vi "Validate Mode.vi"(1 "Mode Array":T1) -> (0 "Mode":i16[](array[numeric]))   [LabVIEW 2019]
uses:
  Version 2/Data Type Defs/Pulse Mode (array).ctl
panel:
  out "Warning":string
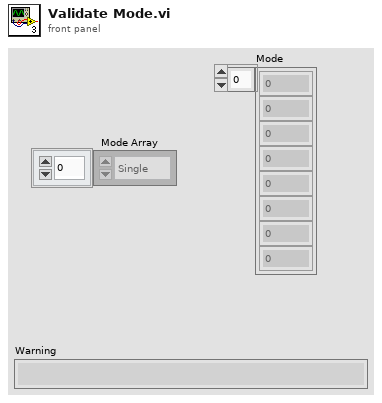
[diagram p1: front panel]
types:
  T1 = typedef "Pulse Mode (array).ctl" = enum16{"Single", "Doublet", "Triplet"}[]
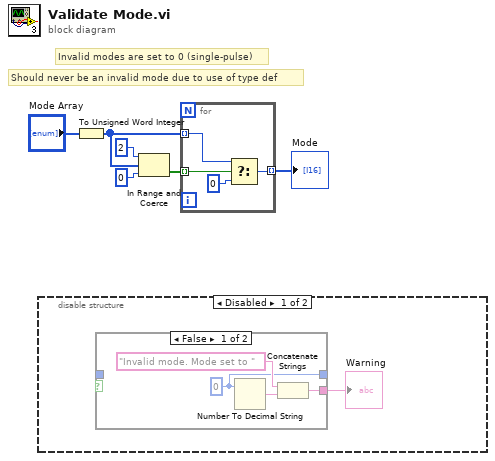
[diagram p0: block diagram]
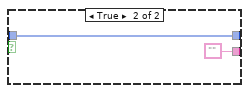
[diagram p2: hidden frame]
diagram:
  # "Should never be an invalid mode due to use of type def"
  # "Invalid modes are set to 0 (single-pulse)"
  n1 = disable-structure shown="Disabled" {
    frame Disabled {
      n2 = case shown="False" {
        selector: _ -> [_ _]
        tunnel: _ -> [_ w12]
        tunnel: [w9 ""] -> w7
        tunnel: [w8 w12] -> _
        frame False {
          w8 = 0
          n3 = Number To Decimal String(number=w8) -> (decimal integer string=w10:string)  [unwired: 1 in]
          n4 = Concatenate Strings("Invalid mode. Mode set to ", w10) -> (w9:string)
        }
        frame True {
        }
      }
      "Warning" <- w7
    }
    frame Enabled {
    }
  }
  n5 = To Unsigned Word Integer(number="Mode Array") -> (unsigned 16bit integer=w2:u16[])
  n6 = In Range and Coerce(upper limit=u16 2, x=w2, lower limit=u16 0) -> (In Range?=w3:bool[])  [unwired: 1 out]
  n7 = for {
    tunnel: w3 -> [w17] mode=indexing
    tunnel: w2 -> [w16] mode=indexing
    tunnel: [w14] -> w1 mode=indexing
    n8 = Select(t=w16, s=w17, f=u16 0) -> (s? t:f=w14:u16)
  }
  "Mode" <- w1
